vi "Update MCL.vi"(8 "error in":errorcluster, 10 "ListBox Refnum":refnum<vi>, 11 "9210 in":refnum<class "9210.lvclass">) -> (0 "error out":errorcluster, 3 "9210 out":refnum<class "9210.lvclass">)   [LabVIEW 2017, in "Modules.lvlib" / "9210.lvclass"]
uses:
  9210.lvclass
  C:/Users/nitest/Documents/NI/niveristand-scan-engine-module-libraries/Source/RSI Module/RSI Module.lvclass
  <vilib>/Utility/miscctls.llb/LVRowAndColumnUnsignedTypeDef.ctl
  9210.lvclass/9210.ctl
  RSI Module/RSI Module.lvclass
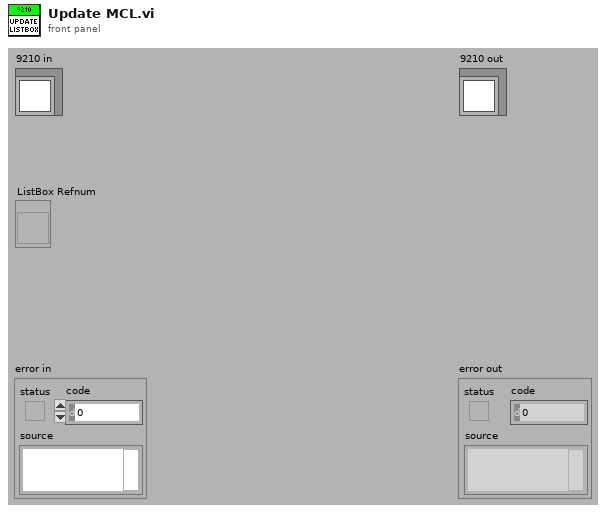
[diagram p1: front panel]
types:
  T1 = typedef "LVRowAndColumnUnsignedTypeDef.ctl" = cluster{"Row":u32, "Column":u32}
  T2 = typedef "Modules.lvlib/RSI Module.lvclass/Channels.ctl" = cluster{"# Input Channels":i32, "# Output Channels":i32, "Channel Type":T3, "Units":string}
  T3 = typedef "Modules.lvlib/RSI Module.lvclass/Channel Type.ctl" = enum16{"Analog", "Digital"}
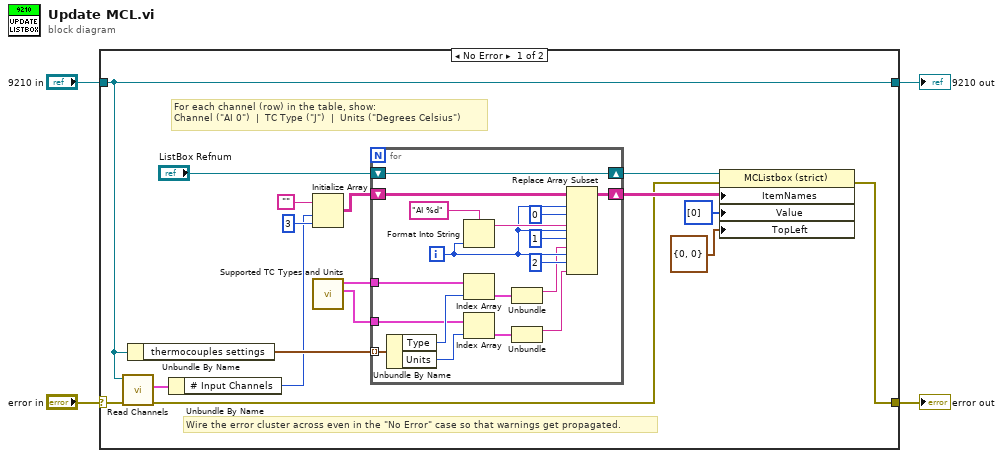
[diagram p0: block diagram]
diagram:
  n1 = case shown="No Error" "error in" {
    selector: "error in" -> [w8 w41]
    tunnel: [w15 w41] -> w3
    tunnel: [w11 w40] -> w1
    tunnel: "9210 in" -> [w11 w40]
    frame No Error {
      # "For each channel (row) in the table, show:\nChannel (\"AI 0\")  |  TC Type (\"J\")  |  Units (\"Degrees Celsius\")"
      # "Wire the error cluster across even in the \"No Error\" case so that warnings get propagated."
      n2 = call "Read Channels.vi"("error in (no error)"=w8, "RSI Module in"=w11) -> ("error out"=w7:errorcluster, "Channels"=w10:T2)  [unwired: 7 in, 1 out]
      n3 = Unbundle By Name(w11) -> ("thermocouples settings"=w12:cluster{"Units":u8, "Type":u8}[])
      n4 = Unbundle By Name(w10) -> ("# Input Channels"=w9:i32)
      n5 = Initialize Array("", w9, 3 ("dimension size")) -> (w18:string[][])
      n6 = call "Supported TC Types and Units.vi"() -> ("supported temperature units"=w6:cluster{"String":string, "Value":u16}[], "supported TC types"=w5:cluster{"String":string, "Value":u16}[])  [unwired: 10 in]
      n7 = for {
        shift-right: [w37] -> w21
        shift-left: w18 -> [w36]
        shift-right: [w39] -> w20
        shift-left: "ListBox Refnum" -> [w39]
        tunnel: w12 -> [w24] mode=indexing
        tunnel: w5 -> [w23]
        tunnel: w6 -> [w22]
        i -> [w33]
        n8 = Unbundle By Name(w24) -> ("Type"=w26:u8, "Units"=w25:u8)
        n9 = Format Into String(format string="AI %d", w33) -> (resulting string=w34:string)  [unwired: 2 in, 1 out]
        n10 = Index Array(array=w23, index=w26) -> (element=w31:cluster{"String":string, "Value":u16})
        n11 = Index Array(array=w22, index=w25) -> (element=w30:cluster{"String":string, "Value":u16})
        n12 = Unbundle(w31) -> ("String"=w28:string)  [unwired: 1 out]
        n13 = Unbundle(w30) -> ("String"=w27:string)  [unwired: 1 out]
        n14 = Replace Array Subset(array=w36, new element #1=w34, index (row) #1=w33, index (col) #1=0 ("Column 1"), new element #2=w28, index (row) #2=w33, index (col) #2=1 ("Column 1"), new element #3=w27, index (row) #3=w33, index (col) #3=2 ("disabled index (col)")) -> (w37:string[][])
      }
      n15 = property on="Property Node" class="MCListbox (strict)"(reference=w20, error in=w7, "ItemNames"=w21, "Value"=i32[] [0], "TopLeft"=T1 {"Row"=0, "Column"=0} ("Top Left Visible Cell")) -> (error out=w15:errorcluster)  [unwired: 1 out]
    }
    frame Error {
    }
  }
  "error out" <- w3
  "9210 out" <- w1
